vi "Offset.vi"(7 "Raw Data Waveform":T1, 10 "Offset":i32, 11 "(Index_Pointer)":refnum<class "Index_Pointer.lvclass">) -> (3 "(Index_Pointer) Out":refnum<class "Index_Pointer.lvclass">)   [LabVIEW 2025, in "Index_Pointer.lvclass"]
uses:
  Index_Pointer.lvclass
  Universal Controls/Waveform_Data.ctl
  Index_Pointer.lvclass/Index_Pointer.ctl
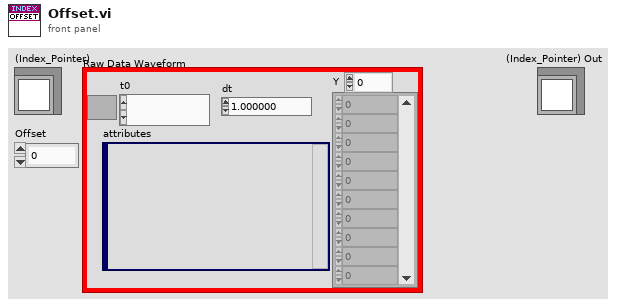
[diagram p1: front panel]
types:
  T1 = typedef "Waveform_Data.ctl" = waveform(dbl)
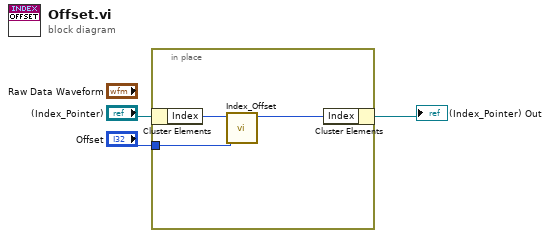
[diagram p0: block diagram]
diagram:
  n1 = in-place {
    in-place-border: "Offset" -> [w4]
    n2 = in-place-cluster #1("(Index_Pointer)") -> ("Index"=w6:i32)
    n3 = call "Index_Offset.vi"("Offset"=w4, "Index"=w6) -> ("Offset Index Out"=w5:i32)  [unwired: 9 in]
    n4 = in-place-cluster #1("Index"=w5) -> (→"(Index_Pointer) Out":refnum<class "Index_Pointer.lvclass">)
  }
